vi "Save-results.vi"(8 "error in (no error)":errorcluster, 10 "Base file path":path, 11 "LaserResponse in":refnum<class "MC-LaserResponse.lvclass">) -> (0 "error out":errorcluster, 1 "Valid?":bool, 3 "LaserResponse":refnum<class "MC-LaserResponse.lvclass">)   [LabVIEW 2013, in "MaterialCharacterization.lvlib" / "MC-LaserResponse.lvclass"]
doc: "Use this template to build a VI to use as a subVI."
uses:
  MC-LaserResponse.lvclass
  MC-LaserResponse.lvclass/MC-LaserResponse.ctl
  <vilib>/Analysis/baseanly.llb/Mean (DBL).vi
  <vilib>/Analysis/NI_AALBase.lvlib
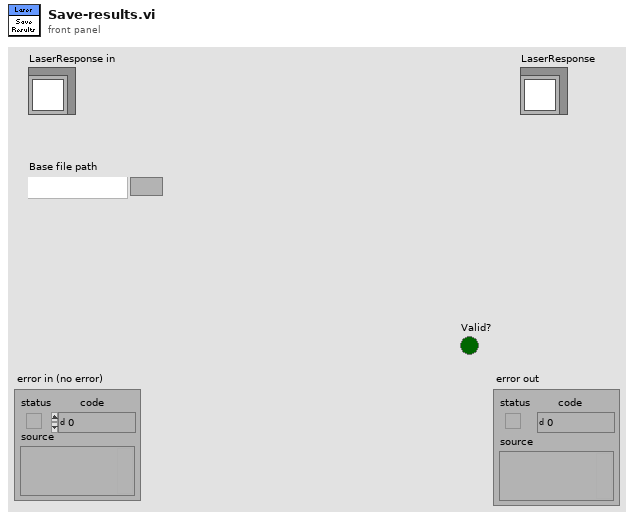
[diagram p1: front panel]
types:
  T1 = enum16{"open", "open or create", "create or replace", "create", "open (read-only)"}
  T2 = enum16{"Undefined", "Modulation (digital)", "Power variation (analog)"}
  T3 = typedef "MaterialCharacterization.lvlib/HC-LaserResponse.lvclass/Detectors.ctl" = enum16{"Undefined", "DET10A", "DET10A - 2kOhm ", "PDA36A - 0dB"}
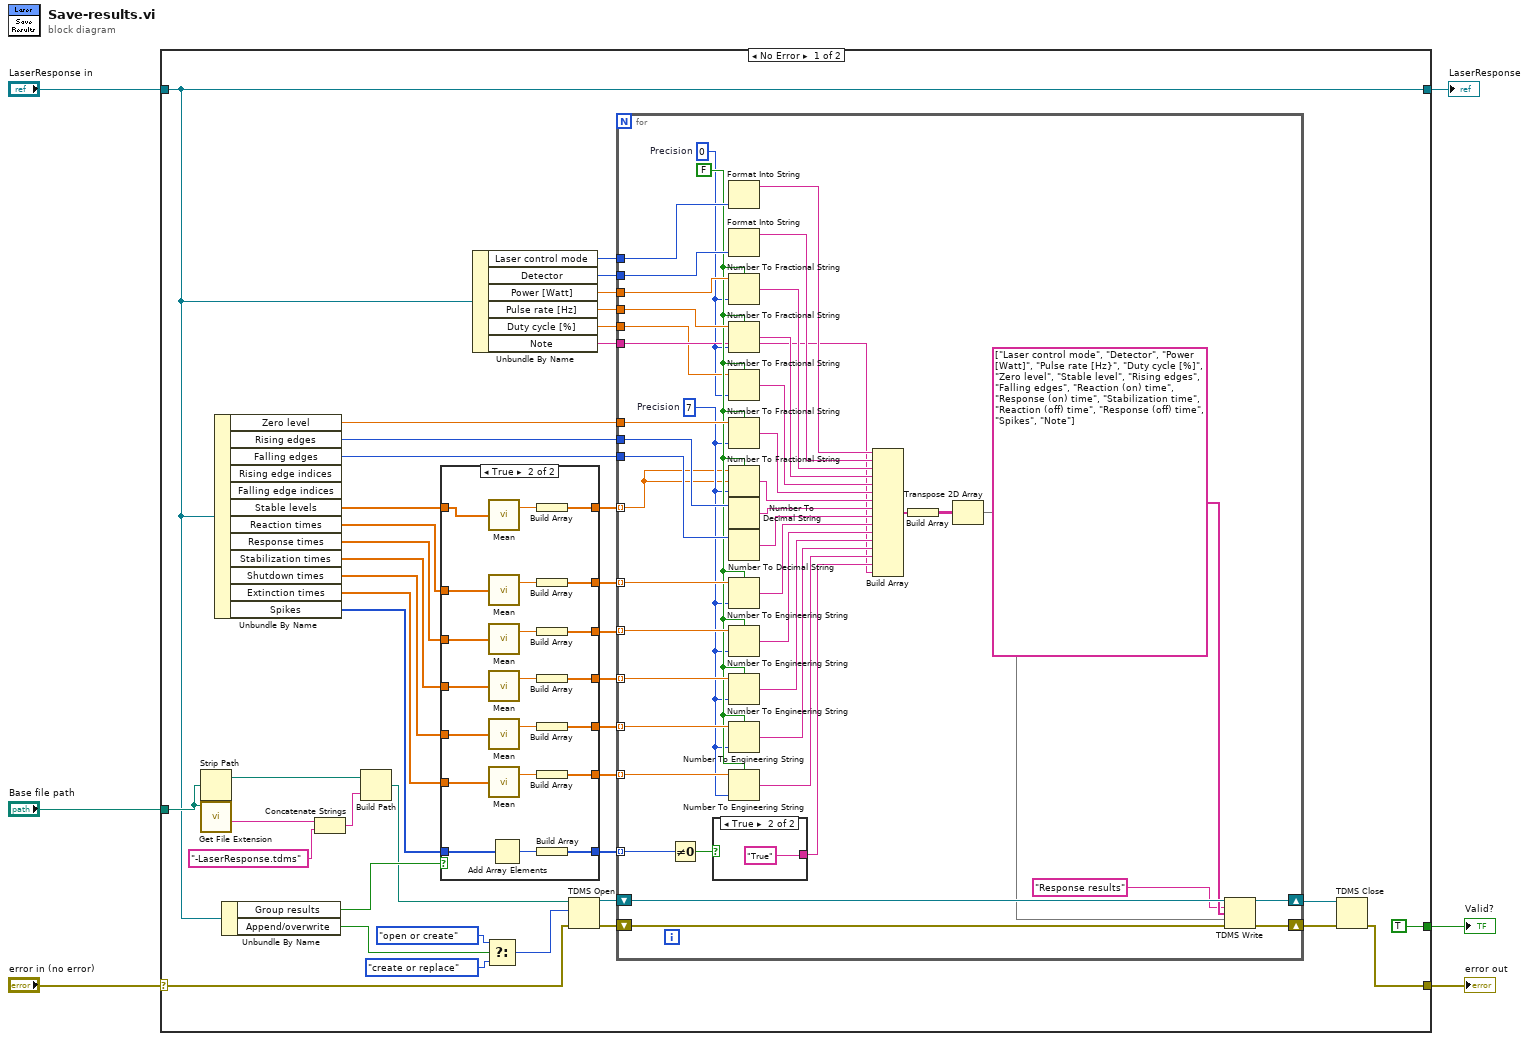
[diagram p0: block diagram]
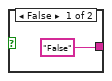
[diagram p3: hidden frame]
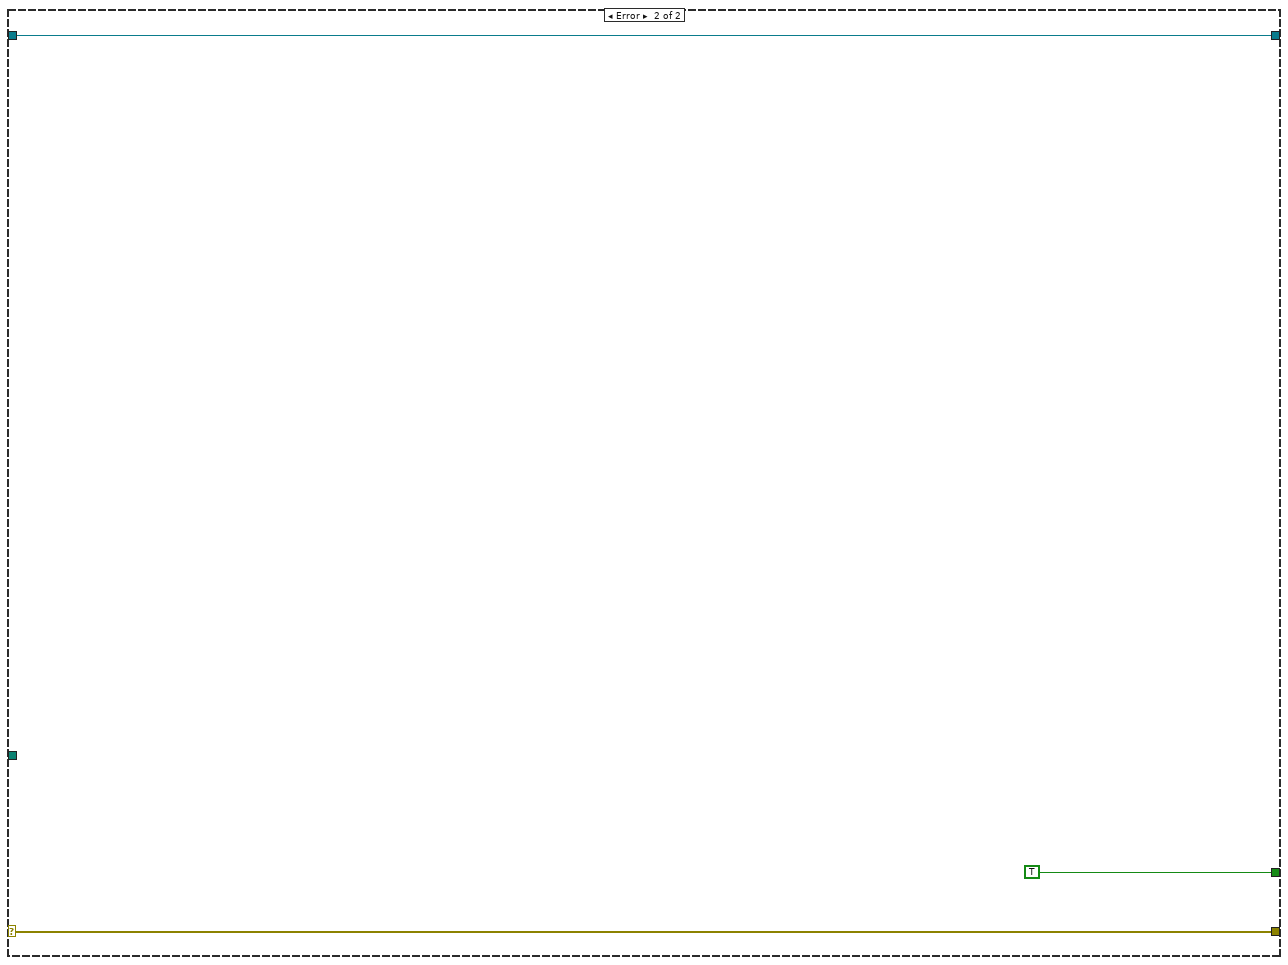
[diagram p4: hidden frame]
diagram:
  n1 = case shown="No Error" "error in (no error)" {
    selector: "error in (no error)" -> [w44 w125]
    tunnel: [w30 w125] -> w5
    tunnel: [TRUE TRUE] -> w4
    tunnel: "LaserResponse in" -> [w9 w123]
    tunnel: [w9 w123] -> w2
    tunnel: "Base file path" -> [w11 _]
    frame No Error {
      n2 = Strip Path(path=w11) -> (stripped path=w15:path)  [unwired: 1 out]
      n3 = call <vilib>:"Get File Extension.vi"("file"=w11) -> ("filename without extension"=w12:string)  [unwired: 7 in, 3 out]
      n4 = Unbundle By Name(w9) -> ("Zero level"=w41:dbl, "Rising edges"=w35:i32, "Falling edges"=w34:i32, "Stable levels"=w8:dbl[], "Reaction times"=w27:dbl[], "Response times"=w26:dbl[], "Stabilization times"=w25:dbl[], "Shutdown times"=w24:dbl[], "Extinction times"=w23:dbl[], "Spikes"=w22:i32[])  [unwired: 2 out]
      n5 = Unbundle By Name(w9) -> ("Group results"=w16:bool, "Append/overwrite"=w45:bool)
      n6 = Concatenate Strings(w12, "-LaserResponse.tdms" ("string")) -> (w14:string)
      n7 = Build Path(base path=w15, name or relative path=w14) -> (appended path=w10:path)
      n8 = case shown="True" w16 {
        tunnel: w27 -> [w55 w76]
        tunnel: [w55 w74] -> w28
        tunnel: w26 -> [w54 w69]
        tunnel: w25 -> [w53 w68]
        tunnel: w24 -> [w52 w67]
        tunnel: w23 -> [w51 w66]
        tunnel: w22 -> [w50 w65]
        tunnel: [w50 w63] -> w21
        tunnel: [w51 w62] -> w20
        tunnel: [w52 w61] -> w19
        tunnel: [w53 w60] -> w18
        tunnel: [w54 w59] -> w17
        tunnel: w8 -> [w49 w57]
        tunnel: [w49 w56] -> w7
        frame False {
        }
        frame True {
          n9 = call-poly <vilib>:"Mean.vi"("X"=w57) -> ("mean"=w58:dbl)  [unwired: 1 out]
          n10 = call-poly <vilib>:"Mean.vi"("X"=w76) -> ("mean"=w75:dbl)  [unwired: 1 out]
          n11 = call-poly <vilib>:"Mean.vi"("X"=w69) -> ("mean"=w73:dbl)  [unwired: 1 out]
          n12 = call-poly <vilib>:"Mean.vi"("X"=w68) -> ("mean"=w72:dbl)  [unwired: 1 out]
          n13 = call-poly <vilib>:"Mean.vi"("X"=w67) -> ("mean"=w71:dbl)  [unwired: 1 out]
          n14 = call-poly <vilib>:"Mean.vi"("X"=w66) -> ("mean"=w70:dbl)  [unwired: 1 out]
          n15 = Add Array Elements(numeric array=w65) -> (sum=w64:i32)
          n16 = Build Array(w58) -> (w56:dbl[])
          n17 = Build Array(w75) -> (w74:dbl[])
          n18 = Build Array(w73) -> (w59:dbl[])
          n19 = Build Array(w72) -> (w60:dbl[])
          n20 = Build Array(w71) -> (w61:dbl[])
          n21 = Build Array(w70) -> (w62:dbl[])
          n22 = Build Array(w64) -> (w63:i32[])
        }
      }
      n23 = Unbundle By Name(w9) -> ("Laser control mode"=w39:T2, "Detector"=w38:T3, "Power [Watt]"=w40:dbl, "Pulse rate [Hz]"=w37:dbl, "Duty cycle [%]"=w36:dbl, "Note"=w33:string)
      n24 = Select(t=T1."open or create" ("operation (0:open)"), s=w45, f=T1."create or replace" ("operation (0:open)")) -> (s? t:f=w48:T1)
      n25 = TDMS Open(8:w44, 10:w48, 11:w10) -> (0:w42:errorcluster, 3:w43:refnum<k34>)  [unwired: 4 in]
      n26 = for {
        tunnel: w41 -> [w117]
        tunnel: w40 -> [w116]
        tunnel: w39 -> [w115]
        tunnel: w38 -> [w114]
        tunnel: w37 -> [w110]
        tunnel: w36 -> [w81]
        tunnel: w35 -> [w105]
        tunnel: w34 -> [w103]
        tunnel: w28 -> [w101] mode=indexing
        tunnel: w17 -> [w100] mode=indexing
        tunnel: w18 -> [w99] mode=indexing
        tunnel: w19 -> [w98] mode=indexing
        tunnel: w20 -> [w96] mode=indexing
        tunnel: w21 -> [w94] mode=indexing
        tunnel: w33 -> [w87]
        shift-right: [w118] -> w31
        shift-left: w42 -> [w119]
        shift-right: [w86] -> w32
        shift-left: w43 -> [w120]
        tunnel: w7 -> [w77] mode=indexing
        w79 = i16 7  # Precision
        w97 = FALSE
        w78 = i16 0  # Precision
        n27 = Not Equal To 0?(x=w94) -> (x != 0?=w95:bool)
        n28 = case shown="True" w95 {
          tunnel: ["False" "True"] -> w88
          frame False {
          }
          frame True {
          }
        }
        n29 = Format Into String(w115) -> (resulting string=w113:string)  [unwired: 3 in, 1 out]
        n30 = Format Into String(w114) -> (resulting string=w112:string)  [unwired: 3 in, 1 out]
        n31 = Number To Fractional String(use system decimal point (T)=w97, number=w116, precision (6)=w78) -> (F-format string=w111:string)  [unwired: 1 in]
        n32 = Number To Fractional String(use system decimal point (T)=w97, number=w110, precision (6)=w78) -> (F-format string=w109:string)  [unwired: 1 in]
        n33 = Number To Fractional String(use system decimal point (T)=w97, number=w81, precision (6)=w78) -> (F-format string=w108:string)  [unwired: 1 in]
        n34 = Number To Fractional String(use system decimal point (T)=w97, number=w117, precision (6)=w79) -> (F-format string=w107:string)  [unwired: 1 in]
        n35 = Number To Fractional String(use system decimal point (T)=w97, number=w77, width (-)=w77, precision (6)=w79) -> (F-format string=w106:string)
        n36 = Number To Decimal String(number=w105) -> (decimal integer string=w104:string)  [unwired: 1 in]
        n37 = Number To Decimal String(number=w103) -> (decimal integer string=w102:string)  [unwired: 1 in]
        n38 = Number To Engineering String(1:w97, 2:w79, 4:w101) -> (0:w93:string)  [unwired: 1 in]
        n39 = Number To Engineering String(1:w97, 2:w79, 4:w100) -> (0:w92:string)  [unwired: 1 in]
        n40 = Number To Engineering String(1:w97, 2:w79, 4:w99) -> (0:w91:string)  [unwired: 1 in]
        n41 = Number To Engineering String(1:w97, 2:w79, 4:w98) -> (0:w90:string)  [unwired: 1 in]
        n42 = Number To Engineering String(1:w97, 2:w79, 4:w96) -> (0:w89:string)  [unwired: 1 in]
        n43 = Build Array(w113, w112, w111, w109, w108, w107, w106, w104, w102, w93, w92, w91, w90, w89, w88, w87) -> (w84:string[])
        n44 = Build Array(w84) -> (w83:string[][])
        n45 = Transpose 2D Array(2D array=w83) -> (transposed array=w80:string[][])
        n46 = TDMS Write(0:w120, 5:"Response results", 7:string[] ["Laser control mode", "Detector", "Power [Watt]", "Pulse rate [Hz}", "Duty cycle [%]", "Zero level", "Stable level", "Rising edges", "Falling edges", "Reaction (on) time", "Response (on) time", "Stabilization time", "Reaction (off) time", "Response (off) time", "Spikes", "Note"], 9:w80, 11:w119) -> (4:w86:refnum<k34>, 15:w118:errorcluster)  [unwired: 1 in, 2 out]
      }
      n47 = TDMS Close(8:w31, 11:w32) -> (0:w30:errorcluster)  [unwired: 1 out]
    }
    frame Error {
    }
  }
  "error out" <- w5
  "Valid?" <- w4
  "LaserResponse" <- w2
